vi "Command_Drive_To_Target.vi"(0 "Startup":bool, 1 "Speed_Y":dbl, 2 "Allowable_Error":dbl=3.0, 3 "Timeout":dbl=3.0) -> (5 "Reinit":bool, 6 "Completed":bool=TRUE, 7 "Speeds":dbl[](array[numeric]))   [LabVIEW 2018]
uses:
  Global_Variables/Sensor_Values.vi
panel:
  in  "Turn Kd":dbl format="%#_13g"
  in  "Turn Ki":dbl format="%#_13g"
  in  "Turn Kp":dbl=0.03 format="%#_13g"
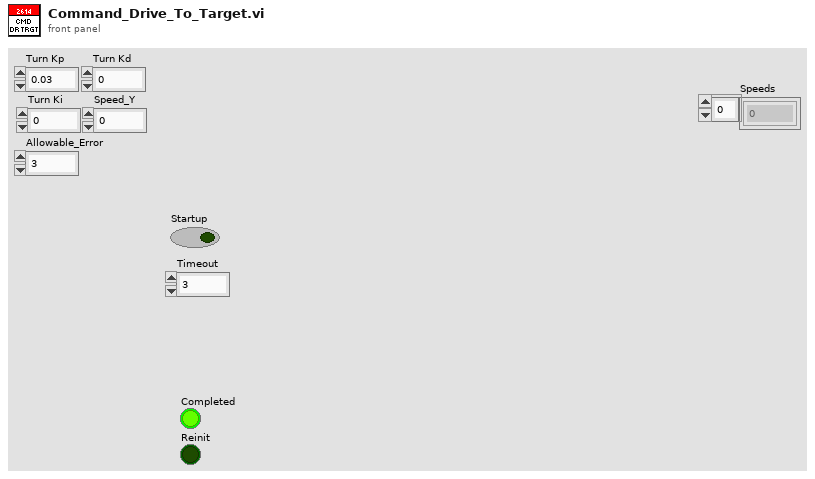
[diagram p1: front panel]
types:
  T1 = cluster{"offsetAngle H":dbl, "offsetAngle V":dbl, "area":dbl, "skew":dbl}
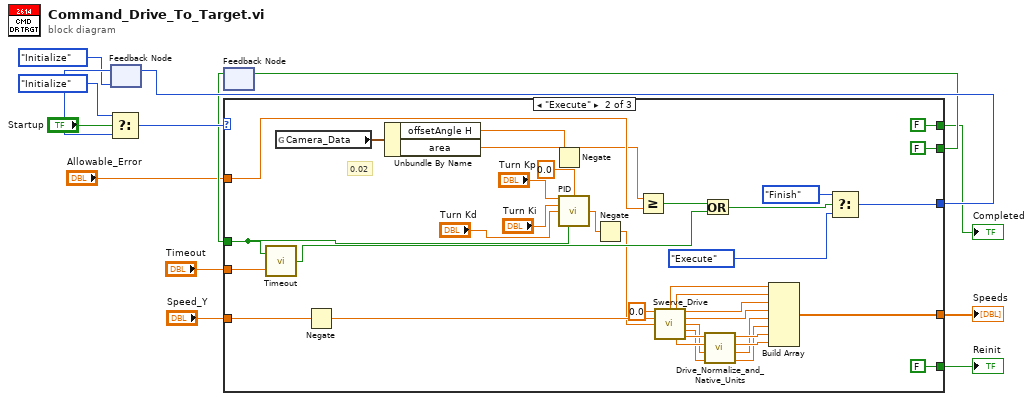
[diagram p0: block diagram]
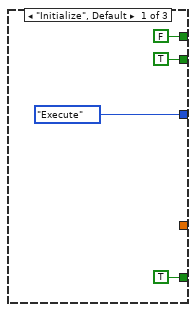
[diagram p2: hidden frame]
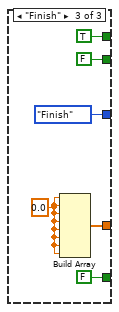
[diagram p3: hidden frame]
diagram:
  n1 = feedback #1(enum16{"Initialize", "Execute", "Finish"}."Initialize" ("f")) -> (w10:enum16{"Initialize", "Execute", "Finish"})
  n2 = Select(t=enum16{"Initialize", "Execute", "Finish"}."Initialize", s="Startup", f=w10) -> (s? t:f=w14:enum16{"Initialize", "Execute", "Finish"})
  n3 = feedback #2() -> (w8:bool)  [unwired: 1 in]
  n4 = case shown="\"Execute\"" w14 {
    tunnel: [enum16{"Initialize", "Execute", "Finish"}."Execute" w53 enum16{"Initialize", "Execute", "Finish"}."Finish" ("f")] -> w11
    tunnel: w8 -> [_ w25 _]
    tunnel: [TRUE FALSE FALSE] -> w9
    tunnel: [FALSE FALSE TRUE] -> w7
    tunnel: [TRUE FALSE FALSE] -> w6
    tunnel: "Timeout" -> [_ w48 _]
    tunnel: [_ w43 w58] -> w3
    tunnel: "Allowable_Error" -> [_ w36 _]
    tunnel: "Speed_Y" -> [_ w26 _]
    frame "Initialize", Default {
    }
    frame "Execute" {
      # "0.02"
      n5 = call "Timeout.vi"("Timeout"=w48, "Initialize"=w25) -> ("Timed Out?"=w49:bool)
      n6 = global read "Sensor_Values.vi" "Camera_Data"() -> (w37:T1)
      n7 = Negate(x=w26) -> (-x=w27:dbl)
      n8 = Unbundle By Name(w37) -> ("offsetAngle H"=w24:dbl, "area"=w22:dbl)
      n9 = Negate(x=w24) -> (-x=w19:dbl)
      n10 = call "PID.vi"("Kp"="Turn Kp", "Process Variable"=w19, "Goal"=0.0, "Ki"="Turn Ki", "Kd"="Turn Kd", "Reinit"=w25) -> ("Command"=w38:dbl)  [unwired: 7 in, 2 out]
      n11 = Negate(x=w38) -> (-x=w21:dbl)
      n12 = Greater Or Equal?(x=w22, y=w36) -> (x >= y?=w39:bool)
      n13 = call "Swerve_Drive.vi"("Z"=0.0, "Y"=w27, "X"=w21) -> ("Back Left Spin Speed"=w47:dbl, "Back Right Spin Speed"=w46:dbl, "Front Left Spin Speed"=w45:dbl, "Front Right Spin Speed"=w44:dbl, "Back Left Motor Power"=w29:dbl, "Back Right Motor Power"=w31:dbl, "Front Right Motor Power"=w35:dbl, "Front Left Motor Power"=w33:dbl)  [unwired: 5 in]
      n14 = Or(x=w39, y=w49) -> (x .or. y?=w50:bool)
      n15 = call "Drive_Normalize_and_Native_Units.vi"("BR"=w31, "BL"=w29, "FR"=w35, "FL"=w33) -> ("BR_Out"=w30:dbl, "BL_Out"=w28:dbl, "FR_Out"=w34:dbl, "FL_Out"=w32:dbl)
      n16 = Build Array(w47, w46, w45, w44, w28, w30, w32, w34) -> (w43:dbl[])
      n17 = Select(t=enum16{"Initialize", "Execute", "Finish"}."Finish", s=w50, f=enum16{"Initialize", "Execute", "Finish"}."Execute") -> (s? t:f=w53:enum16{"Initialize", "Execute", "Finish"})
    }
    frame "Finish" {
      w57 = 0.0 ("element")
      n18 = Build Array(w57, w57, w57, w57, w57, w57, w57, w57) -> (w58:dbl[])
    }
  }
  "Completed" <- w7
  "Reinit" <- w6
  "Speeds" <- w3
  n19 = feedback-in #1(w11) -> ()
  n20 = feedback-in #2(w9) -> ()
